vi "Pade Approximation.vi"(9 "n":i32, 10 "m":i32, 11 "Derivatives":dbl[](array[numeric]) format="%.2f") -> (0 "error":i32, 2 "Denominator":dbl[](array[numeric]) format="%.2f", 3 "Numerator":dbl[](array[numeric]) format="%.2f")   [LabVIEW 2017, in "NI_Gmath.lvlib"]
doc: "Determines the coefficients of a rational polynomial to best suit a given set of derivatives."
uses:
  NI_Gmath.lvlib
  Solve Linear Equations (single right hand).vi
  1D Convolution (DBL).vi
  Solve Linear Equations By Cholesky.vi
  Real Matrix to Compact Array.vi
  Real Compact Tri-Matrix Linear Eqs.vi
  Solve Linear Eqs (General).vi
  Solve Linear Eqs (Gen, single right hand).vi
  NI_AALPro.lvlib
panel:
  # "Example:\n\nDerivatives: (1.3,-2.1,0.3,-2.9,0.1) \nm: 2 \n n: 2"
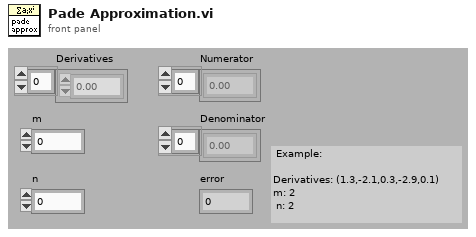
[diagram p1: front panel]
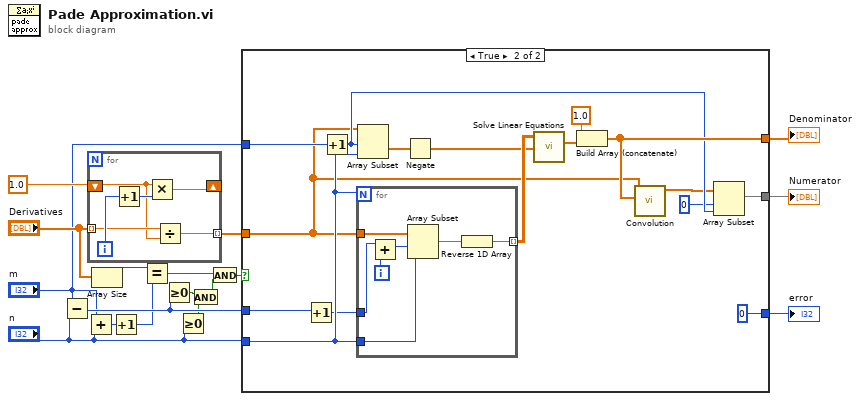
[diagram p0: block diagram]
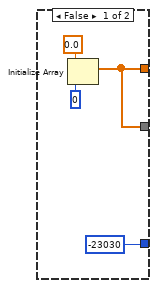
[diagram p2: hidden frame]
diagram:
  n1 = Subtract(x="m", y="n") -> (x-y=w15:i32)
  n2 = Add(x="m", y="n") -> (x+y=w6:i32)
  n3 = for {
    shift-right: [w23] -> _
    shift-left: 1.0 -> [w19]
    tunnel: "Derivatives" -> [w20] mode=indexing
    tunnel: [w18] -> w10 mode=indexing
    i -> [w22]
    n4 = Increment(x=w22) -> (x+1=w21:i32)
    n5 = Multiply(x=w19, y=w21) -> (x*y=w23:dbl)
    n6 = Divide(x=w20, y=w19) -> (x/y=w18:dbl)
  }
  n7 = Array Size(array="Derivatives") -> (size(s)=w2:i32)
  n8 = Increment(x=w6) -> (x+1=w1:i32)
  n9 = Equal?(x=w2, y=w1) -> (x = y?=w5:bool)
  n10 = Greater Or Equal To 0?(x=w15) -> (x >= 0?=w14:bool)
  n11 = Greater Or Equal To 0?(x="n") -> (x >= 0?=w13:bool)
  n12 = And(x=w14, y=w13) -> (x .and. y?=w4:bool)
  n13 = And(x=w5, y=w4) -> (x .and. y?=w3:bool)
  n14 = case shown="True" w3 {
    tunnel: [w25 w43] -> w16
    tunnel: [w25 w42] -> w17
    tunnel: "m" -> [_ w34]
    tunnel: "n" -> [_ w33]
    tunnel: w15 -> [_ w31]
    tunnel: [-23030 0] -> w12
    tunnel: w10 -> [_ w28]
    frame False {
      n15 = Initialize Array(0.0, 0) -> (w25:dbl[])
    }
    frame True {
      n16 = Increment(x=w31) -> (x+1=w32:i32)
      n17 = Increment(x=w34) -> (x+1=w41:i32)
      n18 = for {
        N: w33 -> [_]
        tunnel: w28 -> [w50]
        tunnel: w33 -> [w49]
        tunnel: w32 -> [w48]
        tunnel: [w44] -> w36 mode=indexing
        i -> [w47]
        n19 = Add(x=w48, y=w47) -> (x+y=w46:i32)
        n20 = Array Subset(array=w50, index=w46, length=w49) -> (w45:dbl[])
        n21 = Reverse 1D Array(array=w45) -> (reversed array=w44:dbl[])
      }
      n22 = Array Subset(array=w28, index=w41, length=w33) -> (w35:dbl[])
      n23 = Negate(x=w35) -> (-x=w30:dbl[])
      n24 = call-poly "Solve Linear Equations.vi"("Known Vector"=w30, "Input Matrix"=w36) -> ("Solution Vector"=w37:dbl[])  [unwired: 1 in, 1 out]
      n25 = Build Array (concatenate)(1.0, w37) -> (w43:dbl[])
      n26 = call-poly "Convolution.vi"("Y"=w43, "X"=w28) -> ("X * Y"=w39:dbl[])  [unwired: 8 in, 1 out]
      n27 = Array Subset(array=w39, index=0, length=w41) -> (w42:dbl[])
    }
  }
  "Numerator" <- w17
  "Denominator" <- w16
  "error" <- w12
